vi "Random Number In Range.vi"(1 "하위 리미트":u32, 2 "상위 리미트":u32=1) -> (0 "임의의 수":u32)   [LabVIEW 2010]
doc: "상위 리미트와 하위 리미트로 지정된 범위안에서 임의의 수를 반환합니다."
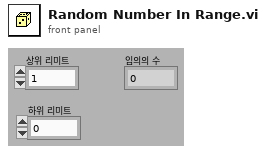
[diagram p1: front panel]
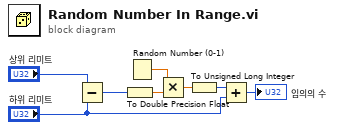
[diagram p0: block diagram]
diagram:
  n1 = Subtract ("빼기")(x="상위 리미트", y="하위 리미트") -> (x-y=w6:u32)
  n2 = To Double Precision Float ("배정도 부동소수로")(number=w6) -> (double precision float=w2:dbl)
  n3 = Random Number (0-1) ("난수(0-1)")() -> (number: 0 to 1=w3:dbl)
  n4 = Multiply ("곱하기")(x=w3, y=w2) -> (x*y=w8:dbl)
  n5 = To Unsigned Long Integer ("부호없는 롱 정수로")(number=w8) -> (unsigned 32bit integer=w1:u32)
  n6 = Add ("더하기")(x=w1, y="하위 리미트") -> (x+y=→"임의의 수":u32)
